vi "GL Set Attribute.vi"(8 "error in":errorcluster, 10 "Value":i32 format="%.0x", 11 "Attribute":T1 items=["SDL_GL_RED_SIZE"=0, "SDL_GL_GREEN_SIZE"=1, "SDL_GL_BLUE_SIZE"=2, "SDL_GL_ALPHA_SIZE"=3, "SDL_GL_BUFFER_SIZE"=4, "SDL_GL_DOUBLEBUFFER"=5, "SDL_GL_DEPTH_SIZE"=6, "SDL_GL_MULTISAMPLEBUFFERS"=13, "SDL_GL_MULTISAMPLESAMPLES"=14]) -> (0 "error out":errorcluster, 3 "Return":i32)   [LabVIEW 2014, in "LibSDL2.lvlib"]
uses:
  LibSDL2.lvlib
  Controls/OpenGL Attribute.ctl
  DLL/SDL2.dll
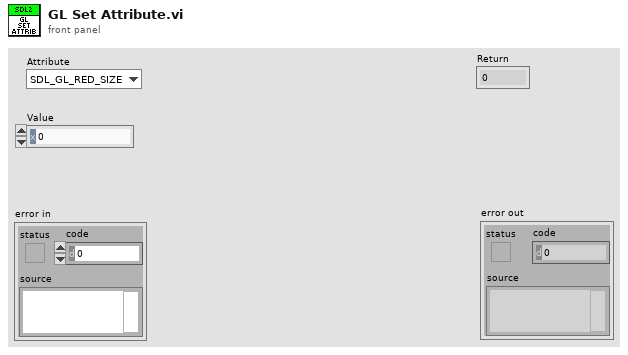
[diagram p1: front panel]
types:
  T1 = typedef "LibSDL2.lvlib/OpenGL Attribute.ctl" = u32
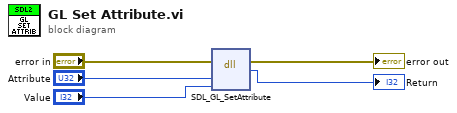
[diagram p0: block diagram]
diagram:
  n1 = dll-call lib="C:/dev/PGS/LabSDL2/Source/LibSDL2 Wrapper/DLL/SDL2.dll" fn="SDL_GL_SetAttribute"(error in="error in", "attribute"="Attribute", "value"="Value") -> (error out=→"error out":errorcluster, "return type"=→"Return":i32)  [unwired: 4 in, 1 out]
